vi "SpectrumVisualizer.vi"(6 "new?":bool=TRUE, 9 "Power":dbl[](array[numeric]), 10 "df":dbl, 11 "f0":dbl) -> (0 "error out":errorcluster)   [LabVIEW 2018, in "lvnetviz.lvlib" / "Spectrum.lvclass"]
uses:
  Spectrum.lvclass
panel:
  in  "Tab Control":enum32{"Traces", "Statistics"}(tab)
  out "Waveform Graph":cluster{"f0":dbl, "df":dbl, "Power":dbl[]}(graph)
  out "Table Control":string[][](table)
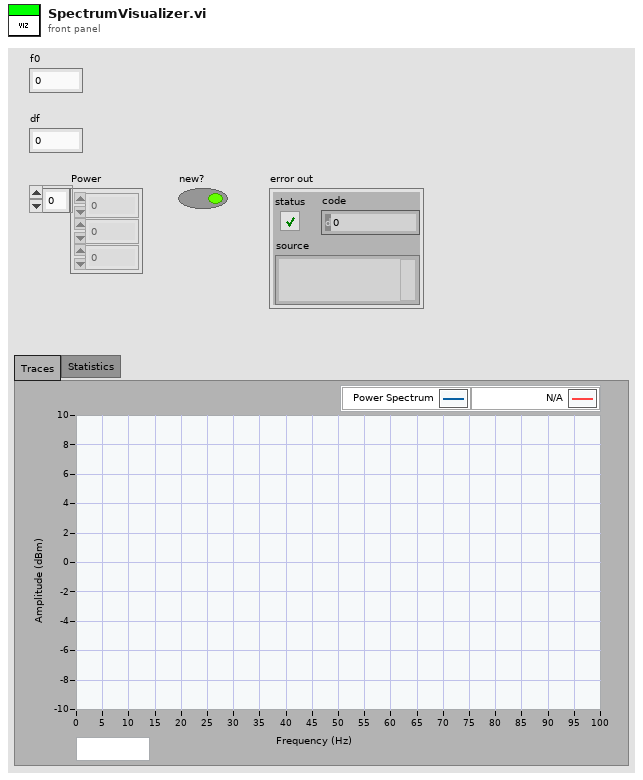
[diagram p1: front panel]
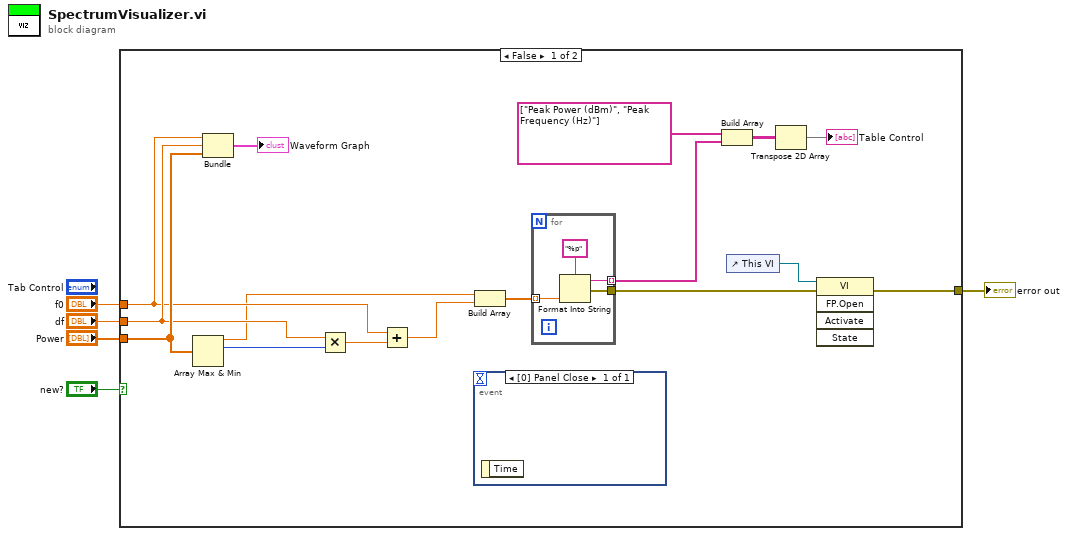
[diagram p0: block diagram]
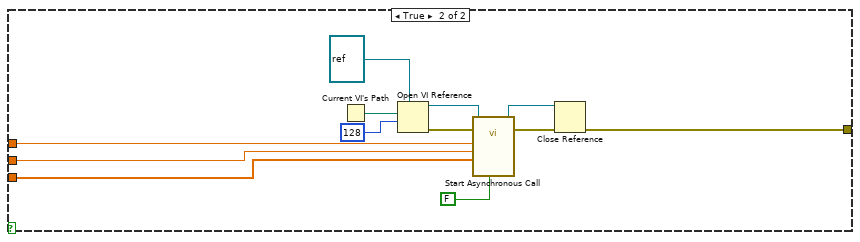
[diagram p2: hidden frame]
diagram:
  n1 = case shown="False" "new?" {
    tunnel: [w8 w29] -> w5
    tunnel: "f0" -> [w17 w26]
    tunnel: "df" -> [w19 w27]
    tunnel: "Power" -> [w20 w28]
    frame False {
      n2 = Array Max & Min(array=w20) -> (max value=w15:dbl, max index (indices)=w16:i32)  [unwired: 2 out]
      n3 = Bundle("f0"=w17, "df"=w19, "Power"=w20) -> (→"Waveform Graph":cluster{"f0":dbl, "df":dbl, "Power":dbl[]})  [unwired: 1 in]
      n4 = Multiply(x=w19, y=w16) -> (x*y=w18:dbl)
      n5 = Add(x=w17, y=w18) -> (x+y=w14:dbl)
      n6 = event shown="[0] Panel Close" {
        selector: _ -> [_]
        dyn-events: _ -> [_]
        timeout: _ -> [_]
        event Panel Close {
          n7 = event-data() -> ()  [unwired: 1 in, 1 out]
        }
      }
      n8 = Build Array(w15, w14) -> (w13:dbl[])
      n9 = for {
        tunnel: [w24] -> w9
        tunnel: w13 -> [w23] mode=indexing
        tunnel: [w22] -> w11 mode=indexing
        n10 = Format Into String(format string="%p", w23) -> (resulting string=w22:string, error out=w24:errorcluster)  [unwired: 2 in]
      }
      n11 = Build Array(string[] ["Peak Power (dBm)", "Peak Frequency (Hz)"], w11) -> (w10:string[][])
      n12 = control-ref of="This VI"() -> (w6:refnum<vi>)
      n13 = Transpose 2D Array(2D array=w10) -> (transposed array=→"Table Control":string[][])
      n14 = invoke class="VI" method="FP.Open"(reference=w6, error in=w9) -> (error out=w8:errorcluster)  [unwired: 3 in, 4 out]
    }
    frame True {
      n15 = Current VI's Path() -> (path=w37:path)
      n16 = Open VI Reference(type specifier VI Refnum (for type only)=refnum<vi> refnum, vi path=w37, options=128) -> (vi reference=w34:refnum<vi>, error out=w32:errorcluster)  [unwired: 3 in]
      n17 = call-by-ref "Start Asynchronous Call"(reference=w34, error in=w32, "new?"=FALSE ("Create New?"), "Power"=w28, "df"=w27, "f0"=w26) -> (reference out=w33:refnum<vi>, error out=w31:errorcluster)  [unwired: 7 in, 1 out]
      n18 = Close Reference(reference=w33, error in (no error)=w31) -> (error out=w29:errorcluster)
    }
  }
  "error out" <- w5
